vi "SQL.Statistic_ProductionStatus.vi"(8 "error in (no error)":errorcluster, 9 "Time":string, 10 "Date":string, 11 "Folder Path":path caption="文件夹路径") -> (0 "error out":errorcluster, 1 "直通率":dbl format="%#_4f", 2 "良品数":u32, 3 "总产量":i32, 4 "XY图":cluster{u32[], u32[]}(graph), 5 "平均时产":dbl)   [LabVIEW 2012, in "Lib_UEL.ATE.lvlib" / "Lib_SQL.lvlib"]
uses:
  Lib_SQL.lvlib
panel:
  out "SQL Results":string[][](table)=[["1.Audio RX", "91.081303", "2.Audio TX", "0.095270", "20121122", "13:32:50", "1170000000689", "PASS"], ["1.Audio RX", "91.143105", "2.Audio TX", "0.095494", "20121122", "13:39:33", "1170000000689", "PASS"], ["1.Audio RX", "91.991153", "2.Audio TX", "0.100831", "20121122", "13:54:04", "1111111111111", "PASS"], ["1.Audio RX", "91.857442", "2.Audio TX", "0.105589", "20121122", "13:56:23", "1172000000041", "PASS"], ["1.Audio RX", "92.085102", "2.Audio TX", "0.101190", "20121122", "13:57:37", "1172000000027", "PASS"], ["1.Audio RX", "91.878361", "2.Audio TX", "0.100191", "20121122", "13:59:11", "1172000000362", "PASS"], ["1.Audio RX", "92.029742", "2.Audio TX", "0.098333", "20121122", "14:02:06", "1172000000287", "PASS"], ["1.Audio RX", "91.480339", "2.Audio TX", "0.101565", "20121122", "14:04:55", "1170000000436", "PASS"], ["1.Audio RX", "91.969090", "2.Audio TX", "0.101169", "20121122", "14:06:27", "1172000000171", "PASS"], ["1.Audio RX", "92.221462", "2.Audio TX", "0.099581", "20121122", "14:09:34", "1172000000034", "PASS"], ["1.Audio RX", "91.987652", "2.Audio TX", "0.098084", "20121122", "14:11:36", "1172000000317", "PASS"], ["1.Audio RX", "92.074553", "2.Audio TX", "0.099366", "20121122", "14:13:21", "1172000000263", "PASS"], ["1.Audio RX", "92.132843", "2.Audio TX", "0.098619", "20121122", "14:14:51", "1172000000492", "PASS"], ["1.Audio RX", "92.082562", "2.Audio TX", "0.099291", "20121122", "14:16:15", "1172000000010", "PASS"], ["1.Audio RX", "91.950055", "2.Audio TX", "0.100073", "20121122", "14:17:31", "1172000000041", "PASS"], ["1.Audio RX", "92.103586", "2.Audio TX", "0.100658", "20121122", "14:28:07", "0000000000000", "PASS"], ["1.Audio RX", "92.130135", "2.Audio TX", "0.099393", "20121122", "14:31:21", "1172000000331", "PASS"], ["1.Audio RX", "92.260601", "2.Audio TX", "0.099085", "20121122", "14:33:09", "1172000000416", "PASS"], ["1.Audio RX", "91.917260", "2.Audio TX", "0.099118", "20121122", "14:34:45", "1172000000294", "PASS"], ["1.Audio RX", "91.905751", "2.Audio TX", "0.097974", "20121122", "14:36:10", "1172000000423", "PASS"], ["1.Audio RX", "92.133605", "2.Audio TX", "0.097918", "20121122", "14:37:41", "1172000000119", "PASS"], ["1.Audio RX", "92.096734", "2.Audio TX", "0.102493", "20121122", "14:40:09", "1172000000508", "PASS"], ["1.Audio RX", "92.042766", "2.Audio TX", "0.097988", "20121122", "14:41:47", "1172000000157", "PASS"], ["1.Audio RX", "92.072530", "2.Audio TX", "0.098405", "20121122", "14:42:41", "1172000000157", "PASS"], ["1.Audio RX", "91.988608", "2.Audio TX", "0.100953", "20121122", "14:45:30", "1172000000164", "PASS"], ["1.Audio RX", "92.115288", "2.Audio TX", "0.099866", "20121122", "14:46:43", "1172000000379", "PASS"], ["1.Audio RX", "91.931552", "2.Audio TX", "0.098401", "20121122", "14:48:07", "1172000000201", "PASS"], ["1.Audio RX", "92.141466", "2.Audio TX", "0.102419", "20121122", "14:49:20", "1172000000324", "PASS"], ["1.Audio RX", "91.932576", "2.Audio TX", "0.099878", "20121122", "14:51:57", "1172000000355", "PASS"], ["1.Audio RX", "92.147045", "2.Audio TX", "0.096185", "20121122", "14:54:23", "1172000000133", "PASS"], ["1.Audio RX", "92.010262", "2.Audio TX", "0.097653", "20121122", "14:55:55", "1172000000270", "PASS"], ["1.Audio RX", "92.200920", "2.Audio TX", "0.099317", "20121122", "14:57:32", "1172000000065", "PASS"], ["1.Audio RX", "92.066286", "2.Audio RX", "91.980270", "20121122", "15:11:29", "", "PASS"], ["1.Audio RX", "92.152783", "2.Audio RX", "92.048697", "20121122", "15:14:00", "", "PASS"], ["1.Audio RX", "92.058673", "2.Audio TX", "0.099819", "20121122", "15:54:48", "1170000000689", "PASS"], ["1.Audio RX", "91.953046", "2.Audio TX", "0.099171", "20121122", "15:58:55", "1170000000436", "PASS"]]
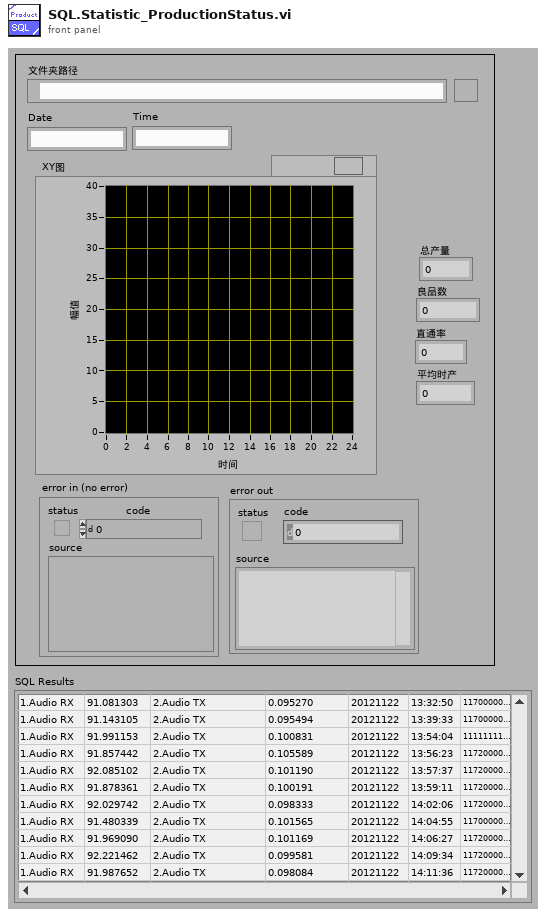
[diagram p1: front panel]
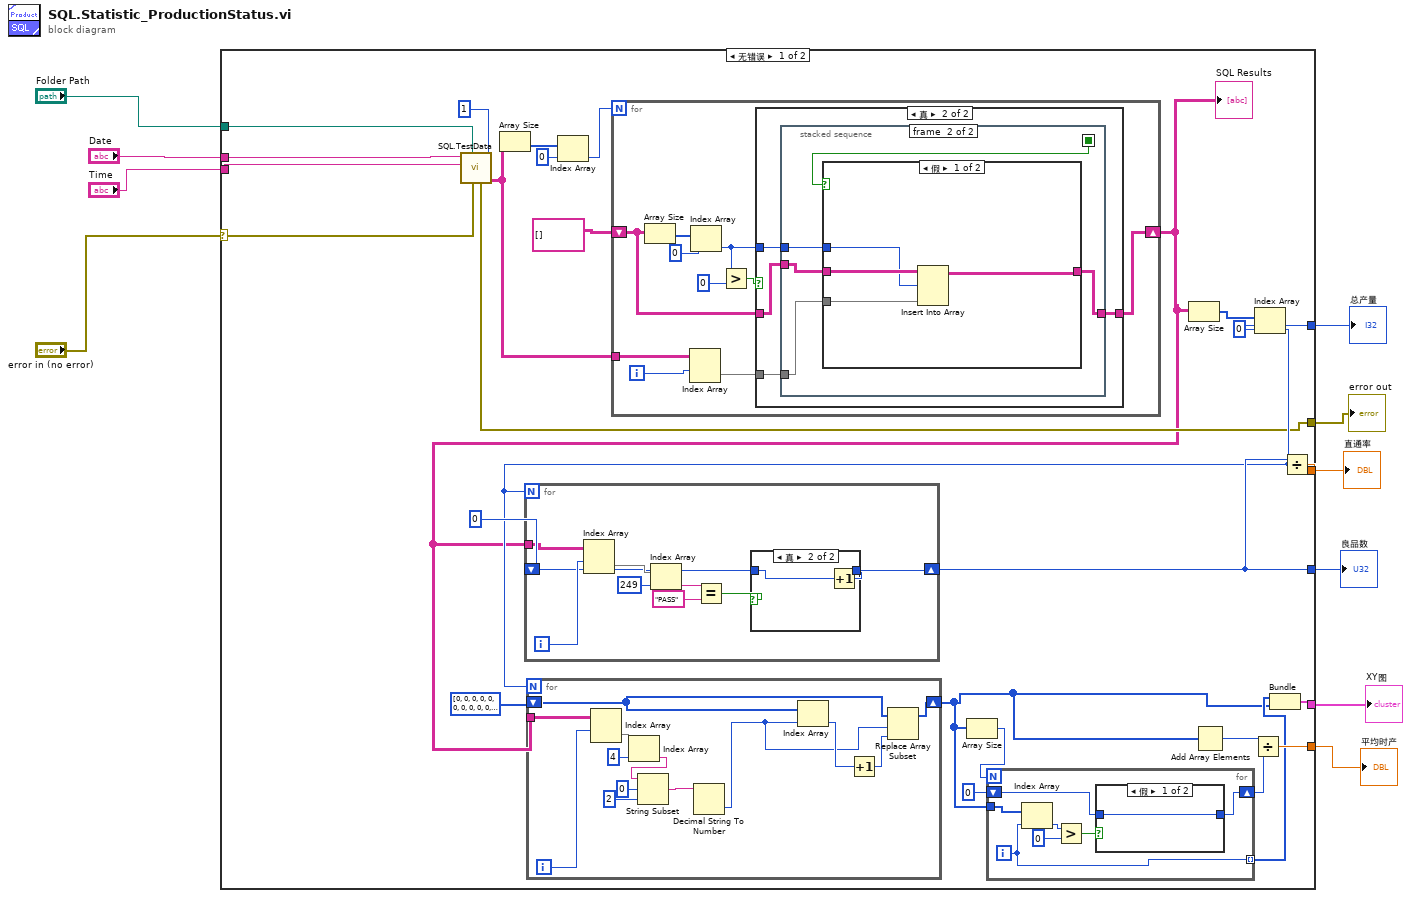
[diagram p0: block diagram]
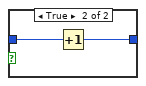
[diagram p2: hidden frame]
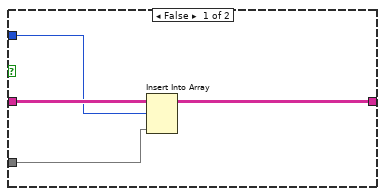
[diagram p4: hidden frame]
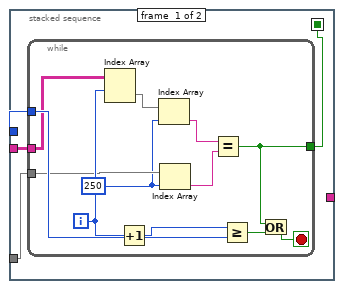
[diagram p5: hidden frame]
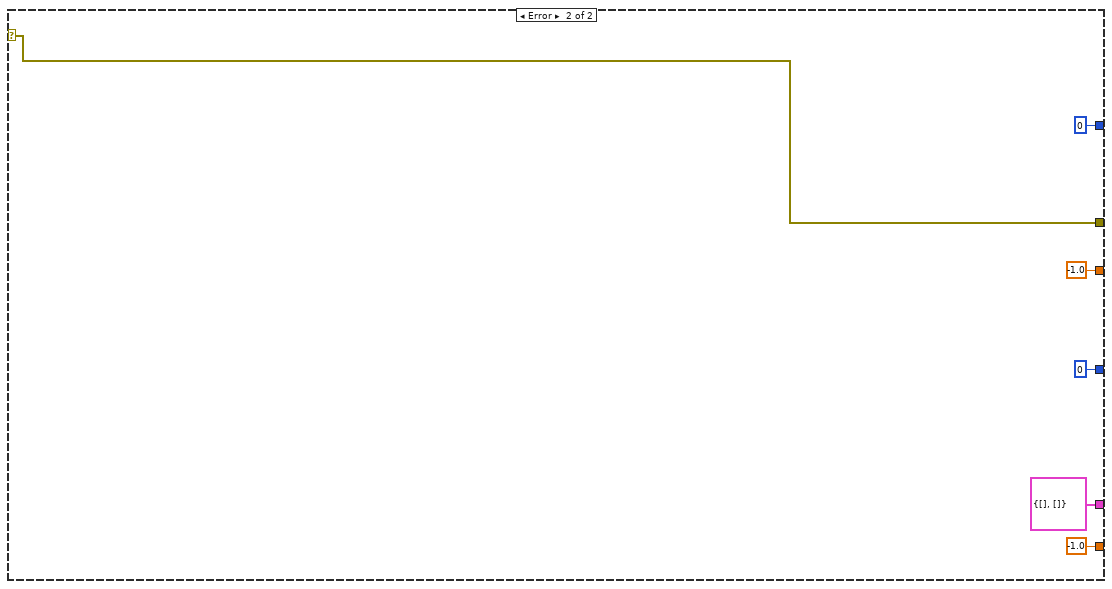
[diagram p7: hidden frame]
diagram:
  n1 = case shown="无错误" "error in (no error)" {
    selector: "error in (no error)" -> [w12 w117]
    tunnel: "Date" -> [w37 _]
    tunnel: "Folder Path" -> [w36 _]
    tunnel: [w27 u32 0 ("良品数")] -> w8
    tunnel: [w26 -1.0] -> w7
    tunnel: [w25 0] -> w6
    tunnel: [w22 -1.0] -> w5
    tunnel: [w21 w117] -> w4
    tunnel: "Time" -> [w20 _]
    tunnel: [w16 cluster{u32[], i32[]} {[], []}] -> w2
    frame No Error {
      n2 = call "SQL.TestData.vi"("最大查询天数"=u32 1, "error in (no error)"=w12, "Folder Path"=w36, "Time"=w20, "Date"=w37) -> ("SQL Results"=w31:string[][], "error out"=w21:errorcluster)  [unwired: 4 in, 1 out]
      n3 = Array Size(array=w31) -> (size(s)=w35:i32[])
      n4 = Index Array(array=w35, index=0 ("索引")) -> (element=w33:i32)
      n5 = for {
        N: w33 -> [_]
        shift-right: [w74] -> w13
        shift-left: string[][] [] ("SQL Results") -> [w78]
        tunnel: w31 -> [w77]
        i -> [w76]
        n6 = Array Size(array=w78) -> (size(s)=w82:i32[])
        n7 = Index Array(array=w77, index (row)=w76) -> (element=w75:string[])  [unwired: 1 in]
        n8 = Index Array(array=w82, index=0 ("索引")) -> (element=w73:i32)
        n9 = Greater?(x=w73, y=0) -> (0:w79:bool)
        n10 = case shown="真" w79 {
          tunnel: w78 -> [w86 w89]
          tunnel: w75 -> [w85 w88]
          tunnel: [w84 w87] -> w74
          tunnel: w73 -> [w83 w90]
          frame False {
            n11 = Insert Into Array(array=w86, index (row)=w83, new element=w85) -> (w84:string[][])  [unwired: 1 in]
          }
          frame True {
            n12 = stacked-sequence {
              seq-local: [w91 _] -> [_ w111]
              tunnel: w90 -> [w94 w107]
              tunnel: w89 -> [w93 w110]
              tunnel: w88 -> [w92 w108]
              tunnel: [_ w109] -> w87
              frame #0 {
                n13 = while {
                  tunnel: w94 -> [w105]
                  tunnel: w93 -> [w102]
                  tunnel: w92 -> [w100]
                  tunnel: [w95] -> w91
                  i -> [w101]
                  stop <- w103 stop-if-true
                  w98 = 250 ("索引")
                  n14 = Index Array(array=w102, index (row)=w101) -> (element=w99:string[])  [unwired: 1 in]
                  n15 = Increment(x=w101) -> (x+1=w106:i32)
                  n16 = Index Array(array=w99, index=w98) -> (element=w97:string)
                  n17 = Index Array(array=w100, index=w98) -> (element=w96:string)
                  n18 = Equal?(x=w97, y=w96) -> (x = y?=w95:bool)
                  n19 = Greater Or Equal?(x=w106, y=w105) -> (x >= y?=w104:bool)
                  n20 = Or(x=w95, y=w104) -> (x .or. y?=w103:bool)
                }
              }
              frame #1 {
                n21 = case shown="假" w111 {
                  tunnel: w110 -> [w115 w116]
                  tunnel: [w113 w116] -> w109
                  tunnel: w108 -> [w114 _]
                  tunnel: w107 -> [w112 _]
                  frame False {
                    n22 = Insert Into Array(array=w115, index (row)=w112, new element=w114) -> (w113:string[][])  [unwired: 1 in]
                  }
                  frame True {
                  }
                }
              }
            }
          }
        }
      }
      "SQL Results" <- w13
      n23 = Array Size(array=w13) -> (size(s)=w30:i32[])
      n24 = Index Array(array=w30, index=0 ("索引")) -> (element=w25:i32)
      n25 = for {
        N: w25 -> [_]
        tunnel: w13 -> [w69]
        shift-right: [w61] -> w27
        shift-left: u32 0 ("良品数") -> [w62]
        i -> [w68]
        n26 = Index Array(array=w69, index (row)=w68) -> (element=w67:string[])  [unwired: 1 in]
        n27 = Index Array(array=w67, index=249 ("索引")) -> (element=w65:string)
        n28 = Equal?(x=w65, y="PASS") -> (x = y?=w63:bool)
        n29 = case shown="真" w63 {
          tunnel: w62 -> [w70 w72]
          tunnel: [w70 w71] -> w61
          frame False {
          }
          frame True {
            n30 = Increment(x=w72) -> (x+1=w71:u32)
          }
        }
      }
      n31 = for {
        N: w25 -> [_]
        tunnel: w13 -> [w60]
        shift-right: [w49] -> w14
        shift-left: u32[] [0, 0, 0, 0, 0, 0, 0, 0, 0, 0, 0, 0, 0, 0, 0, 0, 0, 0, 0, 0, 0, 0, 0, 0] -> [w52]
        i -> [w59]
        n32 = Index Array(array=w60, index (row)=w59) -> (element=w58:string[])  [unwired: 1 in]
        n33 = Index Array(array=w58, index=4 ("索引")) -> (element=w56:string)
        n34 = String Subset(string=w56, offset (0)=0 ("偏移量(0)"), length (rest)=2 ("长度（剩余）")) -> (substring=w53:string)
        n35 = Decimal String To Number(string=w53) -> (number=w48:i32)  [unwired: 2 in, 1 out]
        n36 = Index Array(array=w52, index=w48) -> (element=w51:u32)
        n37 = Increment(x=w51) -> (x+1=w50:u32)
        n38 = Replace Array Subset(array=w52, new element=w50, index=w48) -> (w49:u32[])
      }
      n39 = Array Size(array=w14) -> (size(s)=w19:i32)
      n40 = for {
        N: w19 -> [_]
        tunnel: w14 -> [w44]
        shift-right: [w39] -> w17
        shift-left: u32 0 ("良品数") -> [w40]
        tunnel: [w38] -> w15 mode=indexing
        i -> [w38]
        n41 = Index Array(array=w44, index=w38) -> (element=w43:u32)
        n42 = Greater?(x=w43, y=u32 0) -> (0:w41:bool)
        n43 = case shown="假" w41 {
          tunnel: w40 -> [w45 w47]
          tunnel: [w45 w46] -> w39
          frame False {
          }
          frame True {
            n44 = Increment(x=w47) -> (x+1=w46:u32)
          }
        }
      }
      n45 = Add Array Elements(numeric array=w14) -> (sum=w23:u32)
      n46 = Divide(x=w23, y=w17) -> (x/y=w22:dbl)
      n47 = Bundle(w15, w14) -> (w16:cluster{i32[], u32[]})  [unwired: 1 in]
      n48 = Divide(x=w27, y=w25) -> (x/y=w26:dbl)
    }
    frame Error {
    }
  }
  "直通率" <- w7
  "良品数" <- w8
  "总产量" <- w6
  "平均时产" <- w5
  "error out" <- w4
  "XY图" <- w2
